vi "VoltageScan.vi"() -> ()   [LabVIEW 2016]
uses:
  Input_parameters.ctl
panel:
  in  "Voltage manual range (1.0)":dbl=1.0
  in  "Enable voltage auto range (T:Enable)":bool=TRUE
  in  "Output file":refnum<k7>(container)
  in  "Use source as DMM?":bool
  in  "Scan voltages":string="1\n2\n3"
  out "Current channel":dbl format="%#_13g"
  out "Current voltage (V)":dbl format="%#_13g"
  in  "Data storage location (def: ./results)":path
  in  "AcroPDF":refnum<k7>(container)
  in  "Plot after execution?":bool
  in  "Voltage limit (V)":dbl=1000.0
  in  "Compliance  level (uA)":dbl=10.0
  in  "VISA resource name LCR":refnum<visa-resource-name>
  in  "VISA resource name DMM":refnum<visa-resource-name>
  in  "VISA resource name source":refnum<visa-resource-name>
  in  "Switch delay (s)":dbl=0.01
  in  "Voltage delay (s)":dbl=0.5
  in  "Display channel":i32=1
  in  "Open after execution?":bool
  in  "Identifier":string="test_01"
  in  "Sensor type":enum16{"6''", "8''", "One channel"}(ring)=enum."One channel"
  in  "Measurement type":enum16{"IV", "CV", "Test"}(ring)=enum."Test"
  out "Single channel":cluster{"X":dbl[], "Y":dbl[]}[](graph) caption="XY Graph"
  out "Voltages":cluster{"X":dbl[], "Y":dbl[]}[](graph) caption="XY Graph"
  out "Channels":cluster{i32[], dbl[]}[](graph) caption="XY Graph"
  in  "Stop":bool
  # "Ctrl+H for read mode"
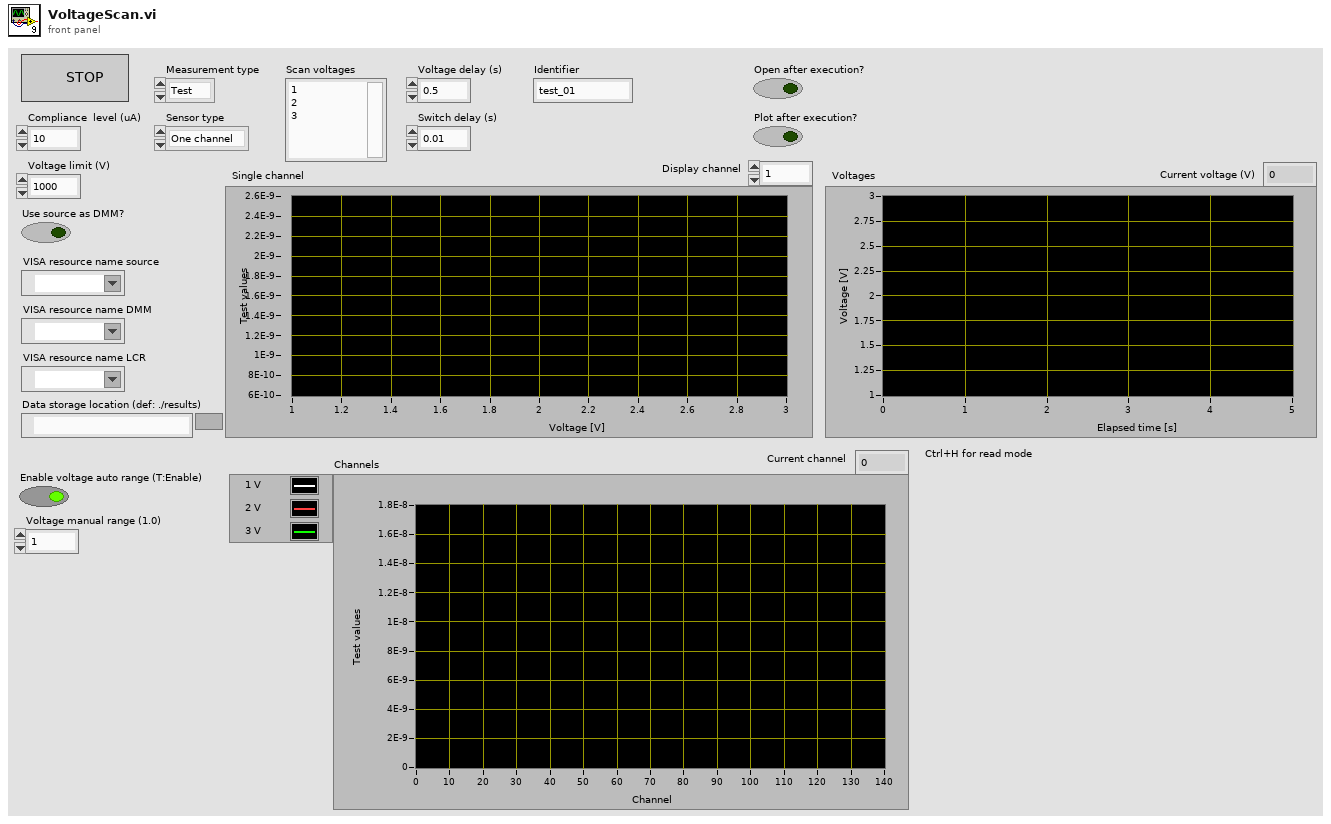
[diagram p1: front panel]
types:
  T1 = typedef "Input_parameters.ctl" = cluster{"Measurement type":enum16{"IV", "CV", "Test"}, "Sensor type":enum16{"6''", "8''", "One channel"}, "Identifier":string, "Open after execution?":bool, "Plot after execution?":bool, "Display channel":i32, "Voltage Delay (s)":dbl, "Switch Delay (s)":dbl, "VISA resource name source":refnum<visa-resource-name>, "VISA resource name DMM":refnum<visa-resource-name>, "VISA resource name LCR":refnum<visa-resource-name>, "Compliance  Level (uA)":dbl, "Voltage Limit (V)":dbl, "Enable Voltage Auto Range (T:Enable)":bool, "Voltage Manual Range (1.0)":dbl, "Data storage location":string, "Scan voltages":string, "Use source as DMM?":bool}
  T2 = typedef "Dynamic_data.ctl" = cluster{"Output file":path, "Y-label text":string, "Current set voltage":dbl, "Voltage column":dbl[], "Pad number column":dbl[], "Data  column":dbl[], "Number of voltages":i32, "Compliance current (A)":dbl, "Geofile":string, "Peak voltage":dbl, "Hex PDF file":string, "Voltage array":dbl[]}
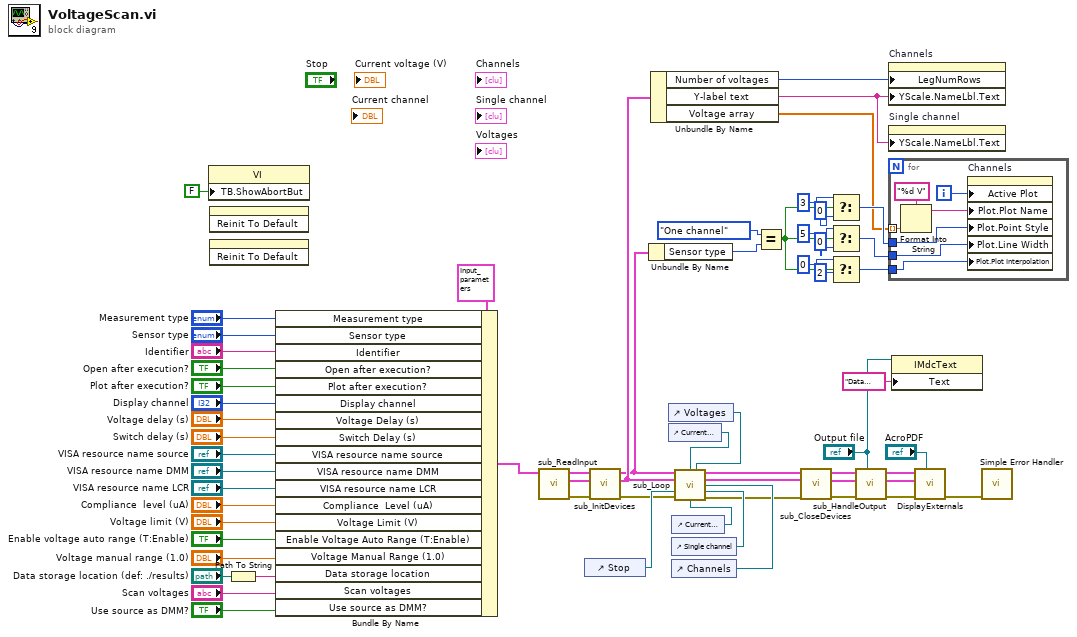
[diagram p0: block diagram]
diagram:
  n1 = property class="VI"("TB.ShowAbortBut"=FALSE ("Tool Bar:Show Abort Button")) -> ()  [unwired: 2 in, 2 out]
  n2 = invoke on="Stop" class="Bool (strict)" method="Reinit To Default"() -> ()  [unwired: 3 in, 3 out]
  n3 = invoke on="Single channel" class="XYGraph (strict)" method="Reinit To Default"() -> ()  [unwired: 3 in, 3 out]
  n4 = Path To String(path="Data storage location (def: ./results)") -> (string=w5:string)
  n5 = Bundle By Name(cluster=T1 {"Measurement type"=enum."Test", "Sensor type"=enum."6''", "Identifier"="test.txt", "Open after execution?"=FALSE, "Plot after execution?"=FALSE, "Display channel"=0, "Voltage Delay (s)"=0.5, "Switch Delay (s)"=0.01, "VISA resource name source"="", "VISA resource name DMM"="", "VISA resource name LCR"="", "Compliance  Level (uA)"=10.0, "Voltage Limit (V)"=1000.0, "Enable Voltage Auto Range (T:Enable)"=TRUE, "Voltage Manual Range (1.0)"=1.0, "Data storage location"="", "Scan voltages"="", "Use source as DMM?"=FALSE} ("Input parameters 2"), "Measurement type"="Measurement type", "Sensor type"="Sensor type", "Identifier"="Identifier", "Open after execution?"="Open after execution?", "Plot after execution?"="Plot after execution?", "Display channel"="Display channel", "Voltage Delay (s)"="Voltage delay (s)", "Switch Delay (s)"="Switch delay (s)", "VISA resource name source"="VISA resource name source", "VISA resource name DMM"="VISA resource name DMM", "VISA resource name LCR"="VISA resource name LCR", "Compliance  Level (uA)"="Compliance  level (uA)", "Voltage Limit (V)"="Voltage limit (V)", "Enable Voltage Auto Range (T:Enable)"="Enable voltage auto range (T:Enable)", "Voltage Manual Range (1.0)"="Voltage manual range (1.0)", "Data storage location"=w5, "Scan voltages"="Scan voltages", "Use source as DMM?"="Use source as DMM?") -> (w21:T1)
  n6 = call "sub_ReadInput.vi"("Input parameters"=w21) -> ("error out"=w61:errorcluster, "Dynamic data"=w58:T2, "Input parameters"=w62:T1)  [unwired: 8 in]
  n7 = control-ref of="Stop"() -> (w54:refnum<vi>)
  n8 = call "sub_InitDevices.vi"("error in (no error)"=w61, "Dynamic data"=w58, "Input parameters"=w62) -> ("error out"=w53:errorcluster, "Dynamic data"=w55:T2, "Input parameters"=w35:T1)  [unwired: 6 in]
  n9 = Unbundle By Name(w35) -> ("Sensor type"=w34:enum16{"6''", "8''", "One channel"})
  n10 = Unbundle By Name(w55) -> ("Number of voltages"=w56:i32, "Y-label text"=w44:string, "Voltage array"=w30:dbl[])
  n11 = control-ref of="Voltages"() -> (w45:refnum<vi>)
  n12 = control-ref of="Current voltage (V)"() -> (w47:refnum<vi>)
  n13 = control-ref of="Current channel"() -> (w46:refnum<vi>)
  n14 = control-ref of="Single channel"() -> (w49:refnum<vi>)
  n15 = control-ref of="Channels"() -> (w50:refnum<vi>)
  n16 = call "sub_Loop.vi"("Input parameters"=w35, "Current voltage"=w47, "Voltages"=w45, "Dynamic data 2"=w55, "Channels"=w50, "Stop"=w54, "Single channel"=w49, "error in (no error)"=w53, "Current channel"=w46) -> ("Input parameters"=w52:T1, "Dynamic data"=w51:T2, "error out"=w48:errorcluster)  [unwired: 4 in]
  n17 = Equal?(x=enum16{"6''", "8''", "One channel"}."One channel" ("Sensor type 2"), y=w34) -> (x = y?=w36:bool)
  n18 = call "sub_CloseDevices.vi"("error in (no error)"=w48, "Dynamic data 2"=w51, "Input parameters"=w52) -> ("error out"=w60:errorcluster, "Dynamic data"=w57:T2, "Input parameters"=w59:T1)  [unwired: 6 in]
  n19 = Select(t=u8 3 ("Plot.Point Style"), s=w36, f=u8 0 ("Plot.Point Style")) -> (s? t:f=w31:u8)
  n20 = Select(t=u8 5 ("Plot.Point Style"), s=w36, f=u8 0 ("Plot.Point Style")) -> (s? t:f=w32:u8)
  n21 = Select(t=u8 0 ("Plot.Point Style"), s=w36, f=u8 2 ("Plot.Point Style")) -> (s? t:f=w33:u8)
  n22 = call "sub_HandleOutput.vi"("Output file text box"="Output file", "error in (no error)"=w60, "Dynamic data 2"=w57, "Input parameters"=w59) -> ("error out"=w28:errorcluster, "Dynamic data"=w27:T2, "Input parameters"=w26:T1)  [unwired: 5 in]
  n23 = property on="Channels" class="XYGraph (strict)"("LegNumRows"=w56, "YScale.NameLbl.Text"=w44) -> ()  [unwired: 2 in, 2 out]
  n24 = property on="Single channel" class="XYGraph (strict)"("YScale.NameLbl.Text"=w44) -> ()  [unwired: 2 in, 2 out]
  n25 = for {
    tunnel: w33 -> [w68]
    tunnel: w32 -> [w67]
    tunnel: w31 -> [w66]
    tunnel: w30 -> [w63] mode=indexing
    i -> [w64]
    n26 = Format Into String(format string="%d V", w63) -> (resulting string=w69:string)  [unwired: 2 in, 1 out]
    n27 = property on="Channels" class="XYGraph (strict)"("Active Plot"=w64, "Plot.Plot Name"=w69, "Plot.Point Style"=w66, "Plot.Line Width"=w67, "Plot.Plot Interpolation"=w68) -> ()  [unwired: 2 in, 2 out]
  }
  n28 = property class="IMdcText"(reference="Output file", "Text"="Data taking in progress...") -> ()  [unwired: 1 in, 2 out]
  n29 = call "DisplayExternals.vi"("AcroPDF"="AcroPDF", "error in (no error)"=w28, "Dynamic data"=w27, "Input parameters"=w26) -> ("error out"=w29:errorcluster)  [unwired: 4 in, 3 out]
  n30 = call <vilib>:"Simple Error Handler.vi"("error in (no error)"=w29) -> ()  [unwired: 4 in, 5 out]
